vi "SerialReadSpeedTest.vi"() -> ()   [LabVIEW 2013]
uses:
  <vilib>/Instr/_visa.llb/VISA Configure Serial Port (Instr).vi
panel:
  out "time dt(ms)":dbl
  in  "t2":dbl
  in  "t1":dbl
  out "output_int16":i32[](array[numeric])
  out "unsigned byte array 2":u8[](array[numeric]) caption="unsigned byte array input"
  in  "stop":bool
  in  "serial_port":refnum<visa-resource-name> caption="Porta Serial"
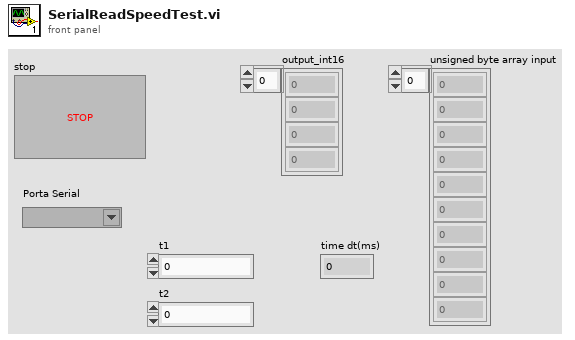
[diagram p1: front panel]
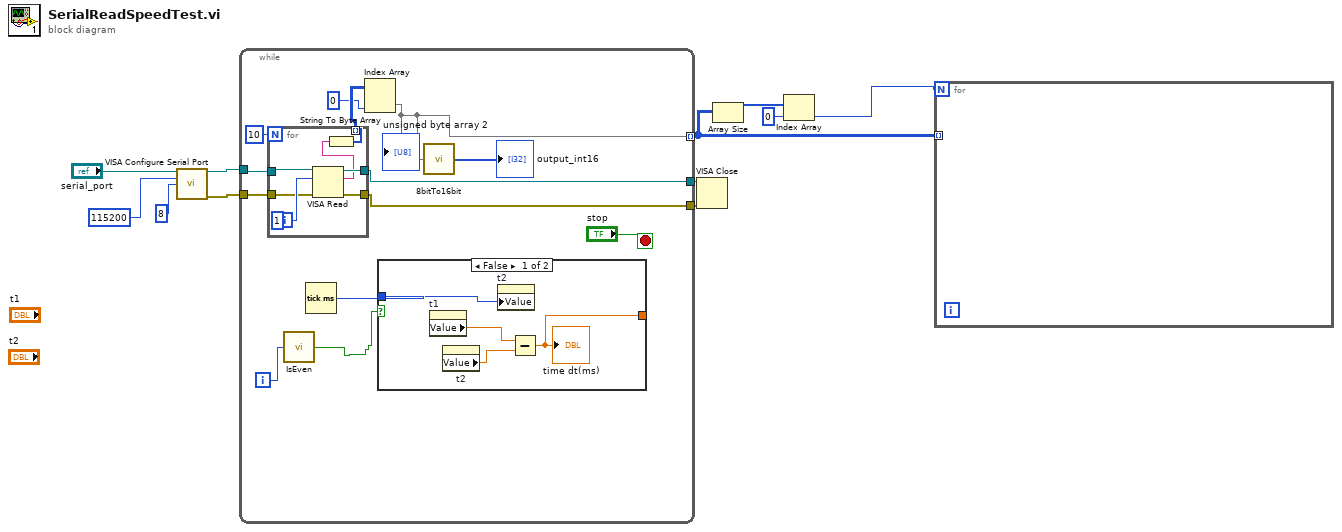
[diagram p0: block diagram]
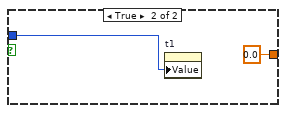
[diagram p2: hidden frame]
diagram:
  n1 = call-poly "VISA Configure Serial Port"("VISA resource name"="serial_port", "baud rate (9600)"=u32 115200, "data bits (8)"=u16 8) -> ("VISA resource name out"=w8:refnum<visa-resource-name>, "error out"=w7:errorcluster)  [unwired: 11 in]
  n2 = while {
    tunnel: w8 -> [w24]
    tunnel: w7 -> [w23]
    tunnel: [w22] -> w6
    tunnel: [w21] -> w5
    tunnel: [w13] -> w4 mode=indexing
    i -> [w17]
    stop <- "stop" stop-if-true
    n3 = for {
      N: 10 -> [_]
      tunnel: w24 -> [w30]
      tunnel: w23 -> [w29]
      tunnel: [w28] -> w22
      tunnel: [w27] -> w21
      tunnel: [w25] -> w14 mode=indexing
      n4 = VISA Read(VISA resource name=w30, byte count=u32 1, error in (no error)=w29) -> (VISA resource name out=w27:refnum<visa-resource-name>, read buffer=w26:string, error out=w28:errorcluster)  [unwired: 1 out]
      n5 = String To Byte Array(string=w26) -> (unsigned byte array=w25:u8[])
    }
    n6 = call "IsEven.vi"("Numeric"=w17) -> ("Boolean"=w16:bool)
    n7 = Tick Count (ms)() -> (millisecond timer value=w18:u32)
    n8 = Index Array(array=w14, index (col)=0 ("index (row)")) -> (element=w13:u8[])  [unwired: 1 in]
    "unsigned byte array 2" <- w13
    n9 = case shown="False" w16 {
      tunnel: w18 -> [w35 w37]
      tunnel: [w32 0.0] -> _
      frame False {
        n10 = property on="t1" class="DigNum (strict)"() -> ("Value"=w34:dbl)  [unwired: 2 in, 2 out]
        n11 = property on="t2" class="DigNum (strict)"() -> ("Value"=w33:dbl)  [unwired: 2 in, 2 out]
        n12 = property on="t2" class="DigNum (strict)"("Value"=w35) -> ()  [unwired: 2 in, 2 out]
        n13 = Subtract(x=w34, y=w33) -> (x-y=w32:dbl)
        "time dt(ms)" <- w32
      }
      frame True {
        n14 = property on="t1" class="DigNum (strict)"("Value"=w37) -> ()  [unwired: 2 in, 2 out]
      }
    }
    n15 = call "8bitTo16bit.vi"("input_byte"=w13) -> ("output_int16"=→"output_int16":i32[])
  }
  n16 = VISA Close(VISA resource name=w5, error in (no error)=w6) -> ()  [unwired: 1 out]
  n17 = Array Size(array=w4) -> (size(s)=w3:i32[])
  n18 = Index Array(array=w3, index=0) -> (element=w1:i32)
  n19 = for {
    N: w1 -> [_]
    tunnel: w4 -> [_] mode=indexing
  }
